vi "3D03_Grab_and_Plot.vi"() -> ()   [LabVIEW 2012]
doc: "The Low-Level Grab Raw Data VI acquires images continuously and displays the images in an image control using low-level acquisition VIs. This VI demonstrates how to acquire raw data from the camera. A grab is appropriate for high-speed applications in which you need to process only one image at a time."
uses:
  <vilib>/userDefined/High Color/IMAQdx.ctl
  <vilib>/vision/driver/IMAQdx.llb/IMAQdx Buffer Number Mode.ctl
  <vilib>/vision/driver/NI_Vision_Acquisition_Software.lvlib
  <resource>/objmgr/imaqdx.rc
  <userlib>/Photonfocus Toolkit/Photonfocus_Toolkit.lvlib
panel:
  out "Linescan Profile":u8[][](array[numeric])
  in  "NumProfiles":u16=700
  out "Width Profile":u8[][](array[numeric])
  out "Quality Profile":u8[][](array[numeric])
  in  "Tab Control":enum32{"Images", "Maps", "3D View"}(tab)
  out "Image":T1(plugin-control)
  out "Peak":sgl[](graph)
  out "Width":u8[](graph)
  out "Quality":u8[](graph)
  out "Range Map":T1(plugin-control)
  out "Width Map":T1(plugin-control)
  out "Quality Map":T1(plugin-control)
  out "Linescan":T1(plugin-control)
  in  "3D Surface":refnum<k7>(container)
  in  "stop":bool
  out "Peak Profile":sgl[][](array[numeric])
  in  "FrameCombine_Enable":bool
  in  "FrameCombine_NrOfFrames":u32
  in  "PeakDetector_Mode":u32
  in  "Camera Name":T2
  out "Buffer Number":u32
  out "Frame Rate":dbl(knob) scale=0.0..100.0 scale format="%.1f"
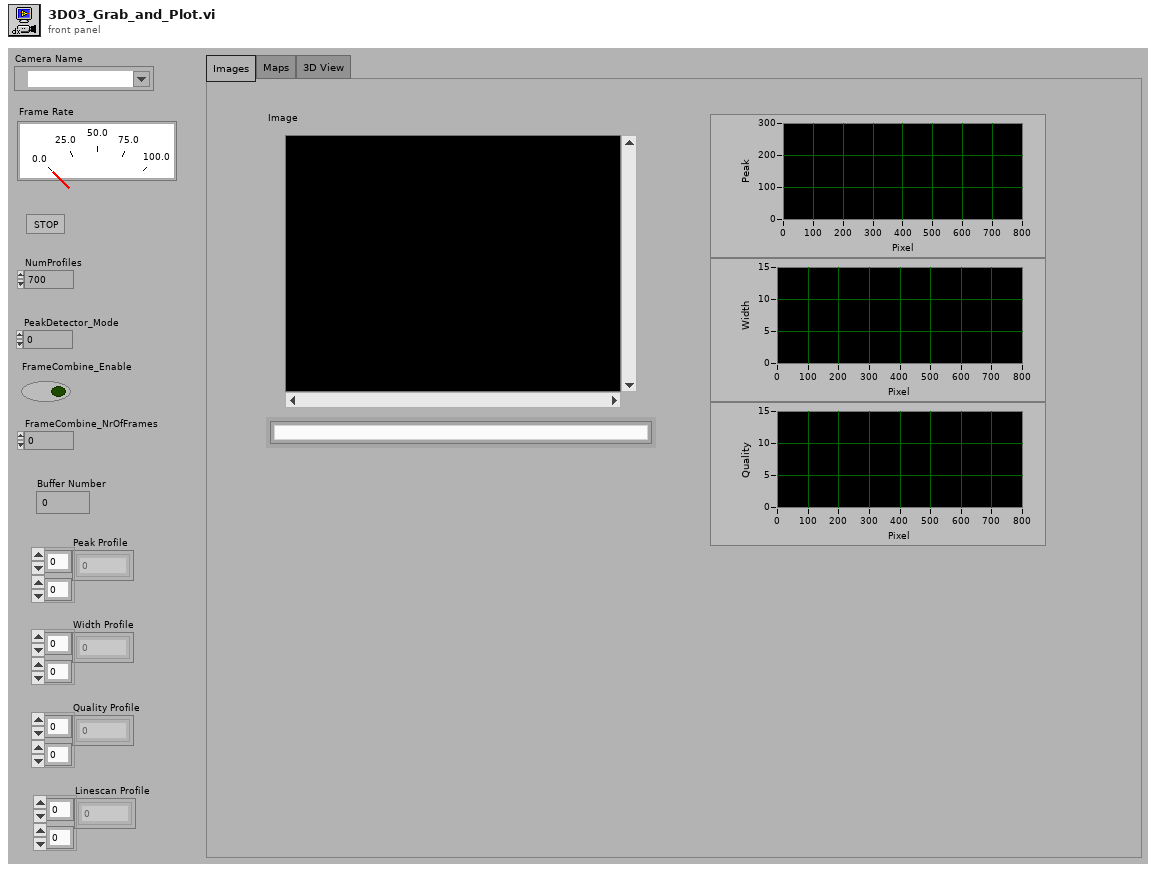
[diagram p1: front panel]
types:
  T1 = typedef "IMAQ Image.ctl" = refnum<image>
  T2 = typedef "IMAQdx.ctl" = refnum<k21>
  T3 = typedef "Image Type" = u32
  T4 = typedef "NI_Vision_Acquisition_Software.lvlib/IMAQdx Buffer Number Mode.ctl" = enum32{"Next", "Last", "Buffer Number"}
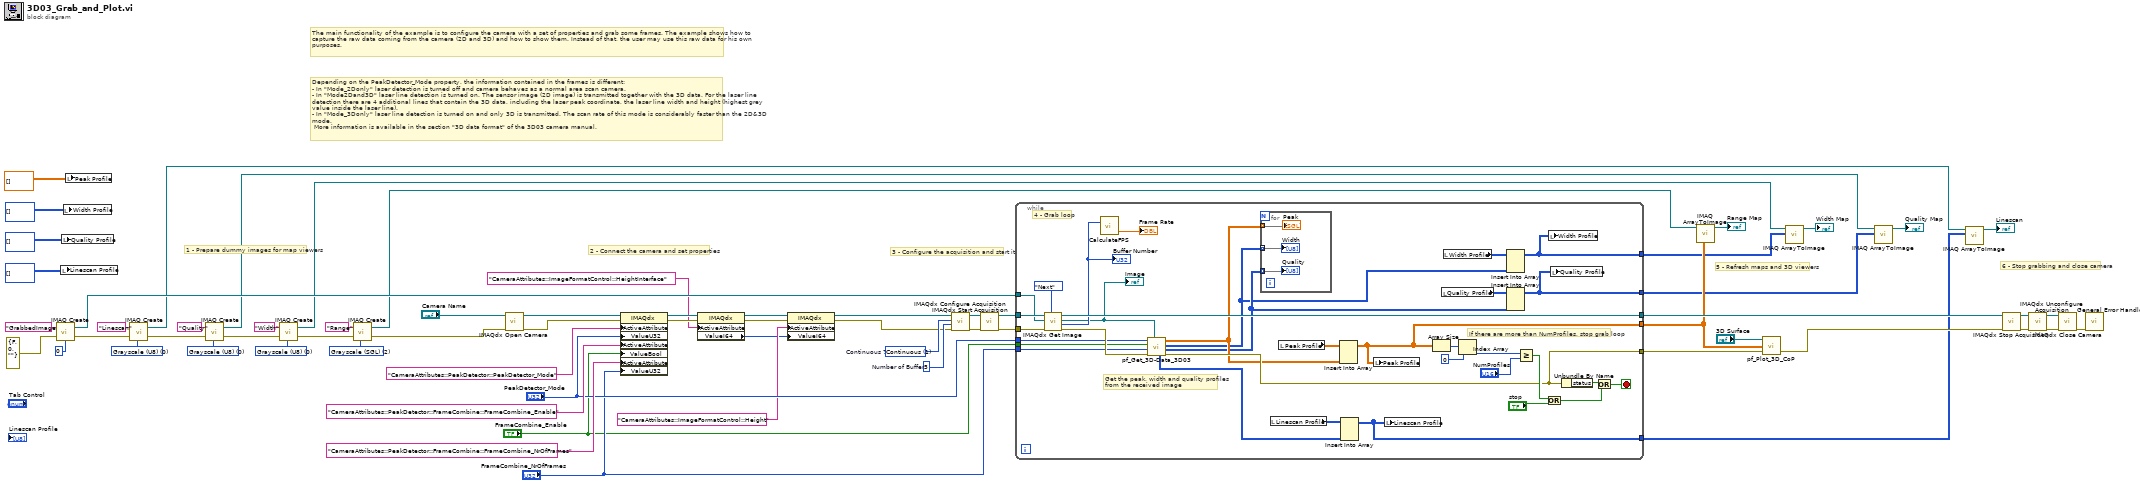
[diagram p0: block diagram]
diagram:
  w7 = T3 0 items=["Grayscale (U8)", "Grayscale (I16)", "Grayscale (SGL)", "Complex (CSG)", "RGB (U32)", "HSL (U32)", "RGB (U64)", "Grayscale (U16)"] ("Image Type")
  w22 = T3 2 items=["Grayscale (U8)", "Grayscale (I16)", "Grayscale (SGL)", "Complex (CSG)", "RGB (U32)", "HSL (U32)", "RGB (U64)", "Grayscale (U16)"] ("Image Type")
  w23 = T3 0 items=["Grayscale (U8)", "Grayscale (I16)", "Grayscale (SGL)", "Complex (CSG)", "RGB (U32)", "HSL (U32)", "RGB (U64)", "Grayscale (U16)"] ("Image Type")
  w33 = T3 0 items=["Grayscale (U8)", "Grayscale (I16)", "Grayscale (SGL)", "Complex (CSG)", "RGB (U32)", "HSL (U32)", "RGB (U64)", "Grayscale (U16)"] ("Image Type")
  w62 = u32 3  # Number of Buffer
  w63 = u32 1 items=["One Shot", "Continuous"]  # Continuous ?
  # "Depending on the PeakDetector_Mode property, the information contained in the frames is different:\n- In \"Mode_2Donly\" laser detection is turned off and camera behaves as a normal area scan camera.\n- In \"Mode2Dand3D\" laser line detection is turned on. The sensor image (2D image) is transmitted together with the 3D data. For the laser line detection there are 4 additional lines that contain the 3D data, including the laser peak coordinate, the laser line width and height (highest grey value inside the laser line).\n- In \"Mode_3Donly\" laser line detection is turned on and only 3D is transmitted. The scan rate of this mode is considerably faster than the 2D&3D mode.\n More information is available in the section \"3D data format\" of the 3D03 camera manual."
  # "The main functionality of the example is to configure the camera with a set of properties and grab some frames. The example shows how to capture the raw data coming from the camera (2D and 3D) and how to show them. Instead of that, the user may use this raw data for his own purposes."
  # "6 - Stop grabbing and close camera"
  # "5 - Refresh maps and 3D viewers"
  # "3 - Configure the acquisition and start it"
  # "2 - Connect the camera and set properties"
  # "1 - Prepare dummy images for map viewers"
  n1 = call "IMAQ Create"("Image Name"="GrabbedImage", "Image Type"=0, "error in (no error)"=errorcluster {"status"=FALSE, "code"=0, "source"=""}) -> ("New Image"=w52:T1, "error out"=w4:errorcluster)  [unwired: 1 in, 1 out]
  n2 = local write "Linescan Profile"(u8[][] []) -> ()
  n3 = local write "Quality Profile"(u8[][] []) -> ()
  n4 = local write "Width Profile"(u8[][] []) -> ()
  n5 = local write "Peak Profile"(dbl[][] []) -> ()
  n6 = call "IMAQ Create"("Image Name"="Linescan", "Image Type"=w7, "error in (no error)"=w4) -> ("New Image"=w3:T1, "error out"=w5:errorcluster)  [unwired: 1 in, 1 out]
  n7 = call "IMAQ Create"("Image Name"="Quality", "Image Type"=w33, "error in (no error)"=w5) -> ("New Image"=w13:T1, "error out"=w21:errorcluster)  [unwired: 1 in, 1 out]
  n8 = call "IMAQ Create"("Image Name"="Width", "Image Type"=w23, "error in (no error)"=w21) -> ("New Image"=w17:T1, "error out"=w26:errorcluster)  [unwired: 1 in, 1 out]
  n9 = call "IMAQ Create"("Image Name"="Range", "Image Type"=w22, "error in (no error)"=w26) -> ("New Image"=w19:T1, "error out"=w20:errorcluster)  [unwired: 1 in, 1 out]
  n10 = call <vilib>:"IMAQdx Open Camera.vi"("error in"=w20, "Session In"="Camera Name") -> ("error out"=w50:errorcluster, "Session Out"=w51:T2)  [unwired: 1 in, 7 out]
  n11 = property class="IMAQdx"(reference=w51, error in=w50, "ActiveAttribute"="CameraAttributes::PeakDetector::PeakDetector_Mode", "ValueU32"="PeakDetector_Mode", "ActiveAttribute"="CameraAttributes::PeakDetector::FrameCombine::FrameCombine_Enable", "ValueBool"="FrameCombine_Enable", "ActiveAttribute"="CameraAttributes::PeakDetector::FrameCombine::FrameCombine_NrOfFrames", "ValueU32"="FrameCombine_NrOfFrames") -> (reference out=w40:T2, error out=w41:errorcluster)
  n12 = property class="IMAQdx"(reference=w40, error in=w41, "ActiveAttribute"="CameraAttributes::ImageFormatControl::HeightInterface") -> (reference out=w39:T2, error out=w42:errorcluster, "ValueI64"=w36:i64)
  n13 = property class="IMAQdx"(reference=w39, error in=w42, "ActiveAttribute"="CameraAttributes::ImageFormatControl::Height", "ValueI64"=w36) -> (reference out=w38:T2, error out=w43:errorcluster)
  n14 = call <vilib>:"IMAQdx Configure Acquisition.vi"("error in"=w43, "Number of Buffers"=w62, "Continuous?"=w63, "Session In"=w38) -> ("error out"=w65:errorcluster, "Session Out"=w64:T2)  [unwired: 6 out]
  n15 = call <vilib>:"IMAQdx Start Acquisition.vi"("error in"=w65, "Session In"=w64) -> ("error out"=w61:errorcluster, "Session Out"=w60:T2)  [unwired: 8 out]
  n16 = while {
    tunnel: [w98] -> w59
    tunnel: w61 -> [w99]
    tunnel: w60 -> [w100]
    tunnel: [w78] -> w30
    tunnel: w52 -> [w94]
    tunnel: "PeakDetector_Mode" -> [w91]
    tunnel: "FrameCombine_Enable" -> [w90]
    tunnel: "FrameCombine_NrOfFrames" -> [w89]
    tunnel: [w76] -> w28
    tunnel: [w71] -> w16
    tunnel: [w70] -> w14
    tunnel: [w67] -> w1
    stop <- w82 stop-if-true
    # "If there are more than NumProfiles, stop grab loop"
    # "Get the peak, width and quality profiles \nfrom the received image"
    # "4 - Grab loop"
    n17 = call <vilib>:"IMAQdx Get Image.vi"("Buffer Number Mode (Next)"=IMAQdx_Buffer_Number_Mode."Next", "error in"=w99, "Image In"=w94, "Session In"=w100) -> ("error out"=w92:errorcluster, "Buffer Number Out"=w95:u32, "Image Out"=w93:T1, "Session Out"=w98:T2)  [unwired: 4 in]
    "Buffer Number" <- w95
    "Image" <- w93
    n18 = call <userlib>:"CalculateFPS.vi"("buffer number"=w95) -> ("processed FPS"=→"Frame Rate":dbl)  [unwired: 2 out]
    n19 = call <userlib>:"pf_Get_3D-Data_3D03.vi"("Aquired Image"=w93, "error in (no error)"=w92, "FrameCombine_NrOfFrames"=w89, "FrameCombine_Enable"=w90, "PealDetector_Mode"=w91) -> ("error out"=w78:errorcluster, "Quality Profile"=w74:u8[][], "Width Profile"=w72:u8[][], "Peak Profile"=w77:sgl[][], "Linescan"=w68:u8[][])  [unwired: 1 in, 1 out]
    n20 = for {
      tunnel: w77 -> [w103] mode=indexing
      tunnel: w72 -> [w102] mode=indexing
      tunnel: w74 -> [w101] mode=indexing
      "Peak" <- w103
      "Width" <- w102
      "Quality" <- w101
    }
    n21 = local read "Linescan Profile"() -> (w69:u8[][])
    n22 = local read "Peak Profile"() -> (w88:sgl[][])
    n23 = Insert Into Array "Insert Into Array"(array=w88, new element=w77) -> (w76:sgl[][])  [unwired: 2 in]
    n24 = Insert Into Array "Insert Into Array"(array=w69, new element=w68) -> (w67:u8[][])  [unwired: 2 in]
    n25 = local write "Peak Profile"(w76) -> ()
    n26 = local write "Linescan Profile"(w67) -> ()
    n27 = Array Size(array=w76) -> (size(s)=w87:i32[])
    n28 = local read "Quality Profile"() -> (w75:u8[][])
    n29 = local read "Width Profile"() -> (w73:u8[][])
    n30 = Index Array(array=w87, index=0) -> (element=w85:i32)
    n31 = Insert Into Array(array=w73, new element=w72) -> (w71:u8[][])  [unwired: 2 in]
    n32 = Insert Into Array(array=w75, new element=w74) -> (w70:u8[][])  [unwired: 2 in]
    n33 = Greater Or Equal?(x=w85, y="NumProfiles") -> (x >= y?=w79:bool)
    n34 = Or(x=w79, y="stop") -> (x .or. y?=w81:bool)
    n35 = local write "Width Profile"(w71) -> ()
    n36 = local write "Quality Profile"(w70) -> ()
    n37 = Unbundle By Name(w78) -> ("status"=w83:bool)
    n38 = Or(x=w83, y=w81) -> (x .or. y?=w82:bool)
  }
  n39 = call "IMAQ ArrayToImage"("Image Pixels (Float)"=w28, "Image"=w19) -> ("Image Out"=→"Range Map":T1)  [unwired: 4 in, 5 out]
  n40 = call <userlib>:"pf_Plot_3D_CoP.vi"("error in (no error)"=w30, "Range Map in"=w28, "3D Surface"="3D Surface") -> ("error out"=w29:errorcluster)  [unwired: 2 in]
  n41 = call "IMAQ ArrayToImage"("Image Pixels (U8)"=w16, "Image"=w17) -> ("Image Out"=→"Width Map":T1)  [unwired: 4 in, 5 out]
  n42 = call "IMAQ ArrayToImage"("Image Pixels (U8)"=w14, "Image"=w13) -> ("Image Out"=→"Quality Map":T1)  [unwired: 4 in, 5 out]
  n43 = call "IMAQ ArrayToImage"("Image Pixels (U8)"=w1, "Image"=w3) -> ("Image Out"=→"Linescan":T1)  [unwired: 4 in, 5 out]
  n44 = call <vilib>:"IMAQdx Stop Acquisition.vi"("error in"=w29, "Session In"=w59) -> ("error out"=w58:errorcluster, "Session Out"=w57:T2)  [unwired: 8 out]
  n45 = call <vilib>:"IMAQdx Unconfigure Acquisition.vi"("error in"=w58, "Session In"=w57) -> ("error out"=w55:errorcluster, "Session Out"=w56:T2)  [unwired: 8 out]
  n46 = call <vilib>:"IMAQdx Close Camera.vi"("error in"=w55, "Session In"=w56) -> ("error out"=w66:errorcluster)  [unwired: 9 out]
  n47 = call <vilib>:"General Error Handler.vi"("error in (no error)"=w66) -> ()  [unwired: 1 in, 14 out]
